vi "Curtin1_NotesDialog.vi"(11 "Files":T1[](array[typedef])) -> (0 "Color":u32[](array[colorbox]), 2 "removed?":bool, 3 "Array":T1[](array[typedef]))   [LabVIEW 2022 SP3]
uses:
  Curtin1_Label.ctl
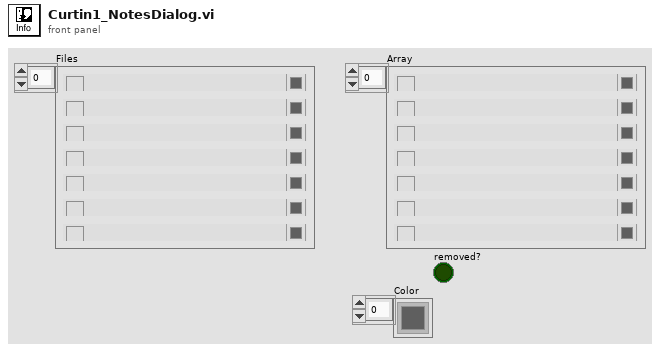
[diagram p1: front panel]
types:
  T1 = typedef "Curtin1_Label.ctl" = cluster{"Show?":bool, "Name":string, "Color":u32, "Path":path, "Show Notes":bool}
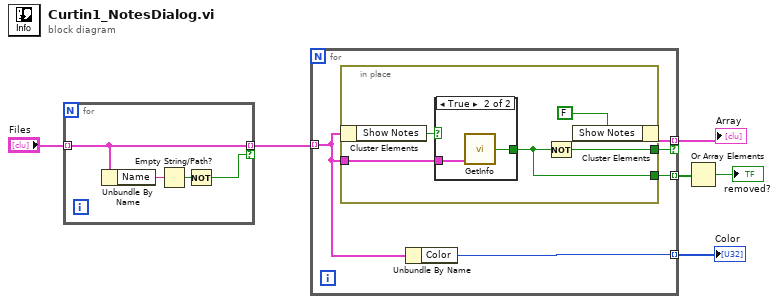
[diagram p0: block diagram]
diagram:
  n1 = for {
    tunnel: "Files" -> [w9] mode=indexing
    tunnel: [w9] -> w3 mode=indexing if=w7
    n2 = Unbundle By Name(w9) -> ("Name"=w10:string)
    n3 = Empty String/Path?(string/path=w10) -> (empty?=w8:bool)
    n4 = Not(x=w8) -> (.not. x?=w7:bool)
  }
  n5 = for {
    tunnel: w3 -> [w14] mode=indexing
    tunnel: [w15] -> w6 mode=indexing if=w12
    tunnel: [w13] -> w5 mode=indexing
    tunnel: [w11] -> w2 mode=indexing
    n6 = in-place {
      in-place-border: w14 -> [w18]
      in-place-border: [w17] -> w12
      in-place-border: [w16] -> w11
      n7 = in-place-cluster #1(w14) -> ("Show Notes"=w20:bool)
      n8 = case shown="True" w20 {
        tunnel: w18 -> [_ w22]
        tunnel: [_ w21] -> w16
        frame False {
        }
        frame True {
          n9 = call "GetInfo.vi"("File selected"=w22) -> ("remove?"=w21:bool)  [unwired: 10 in]
        }
      }
      n10 = Not(x=w16) -> (.not. x?=w17:bool)
      n11 = in-place-cluster #1("Show Notes"=FALSE) -> (w15:T1)
    }
    n12 = Unbundle By Name(w14) -> ("Color"=w13:u32)
  }
  "Array" <- w6
  "Color" <- w5
  n13 = Or Array Elements(Boolean array=w2) -> (logical OR=→"removed?":bool)
